vi "read ring control values and indexes.vi"(7 "error in (no error)":errorcluster, 10 "Ring Ref":refnum<vi>[](array[refnum])) -> (0 "error out":errorcluster, 2 "values & indexes":string[](array[string]))   [LabVIEW 2024]
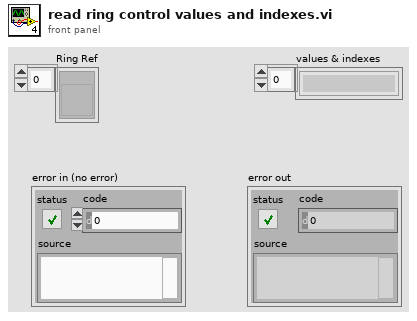
[diagram p1: front panel]
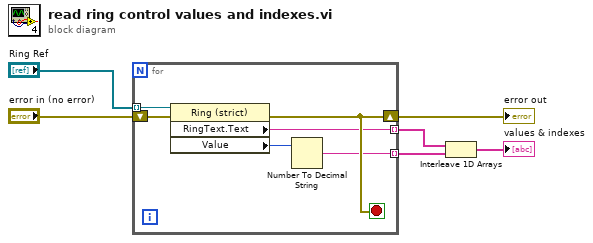
[diagram p0: block diagram]
diagram:
  n1 = for {
    tunnel: "Ring Ref" -> [w11] mode=indexing
    tunnel: [w9] -> w4 mode=indexing
    tunnel: [w8] -> w5 mode=indexing
    shift-right: [w12] -> w3
    shift-left: "error in (no error)" -> [w7]
    stop <- w12 stop-if-true
    n2 = property class="Ring (strict)"(reference=w11, error in=w7) -> (error out=w12:errorcluster, "RingText.Text"=w9:string, "Value"=w10:u16)  [unwired: 1 out]
    n3 = Number To Decimal String(number=w10) -> (decimal integer string=w8:string)  [unwired: 1 in]
  }
  "error out" <- w3
  n4 = Interleave 1D Arrays(w4, w5) -> (→"values & indexes":string[])
